vi "Manual Control - Displacement (SubVI).vi"(0 "Digital in":refnum<vi>, 2 "Disp name":string, 3 "error in (no error)":errorcluster) -> (7 "Numeric":dbl, 10 "error out":errorcluster)   [LabVIEW 2019]
uses:
  Controls/FGV States.ctl
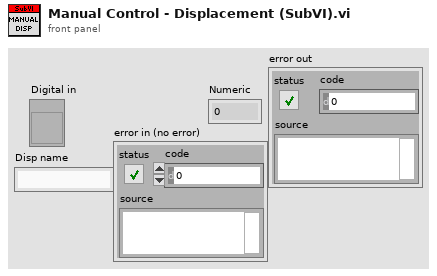
[diagram p1: front panel]
types:
  T1 = typedef "FGV States.ctl" = enum16{"Read", "Write"}
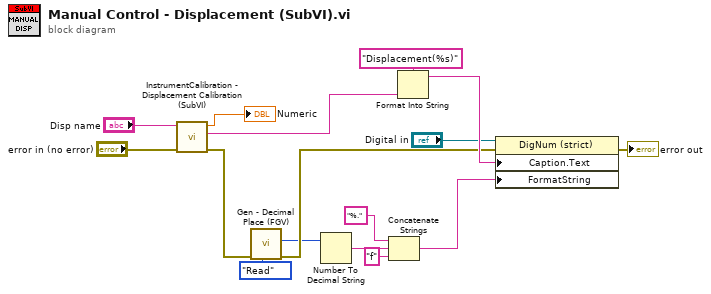
[diagram p0: block diagram]
diagram:
  n1 = call "InstrumentCalibration - Displacement Calibration (SubVI).vi"("error in (no error)"="error in (no error)", "Motor No"="Disp name") -> ("error out"=w4:errorcluster, "Unit"=w7:string, "Displacement"=→"Numeric":dbl)  [unwired: 6 in, 1 out]
  n2 = call "Gen - Decimal Place (FGV).vi"("Action"=FGV_States."Read", "error In"=w4) -> ("error out"=w3:errorcluster, "Ch2 out"=w1:u8)  [unwired: 7 in, 1 out]
  n3 = Number To Decimal String(number=w1) -> (decimal integer string=w13:string)  [unwired: 1 in]
  n4 = Concatenate Strings("%." ("Format String"), w13, "f" ("string")) -> (w9:string)
  n5 = Format Into String(format string="Displacement(%s)" ("initial string"), w7) -> (resulting string=w16:string)  [unwired: 2 in, 1 out]
  n6 = property on="Property Node" class="DigNum (strict)"(reference="Digital in", error in=w3, "Caption.Text"=w16, "FormatString"=w9) -> (error out=→"error out":errorcluster)  [unwired: 1 out]
